vi "CLD3 FGV Timer Solution.vi"(8 "Fehler (Eingang)":T1, 10 "Zielzeit (s)":dbl, 11 "Timer-Modus":T2) -> (0 "Fehler (Ausgang)":T1, 2 "Zeit ist verstrichen":bool, 3 "Verstrichene Zeit (s,ms)":dbl format="%#.2f")   [LabVIEW 2009]
doc: "CLD-Übung 3\nDieses VI wird als FGV zum Messen von Zeit verwendet. \nHinweis zum Auslesen der Zeit während der Pause. Der Entwickler sollte die Funktion \"Zeit lesen\" nicht während der Pause aufrufen. Mit Hilfe einer Case-Struktur kann \"Status abfragen\" jedoch präventiv für diese Möglichkeit programmiert werden."
uses:
  CLD3 FGV Mode.ctl
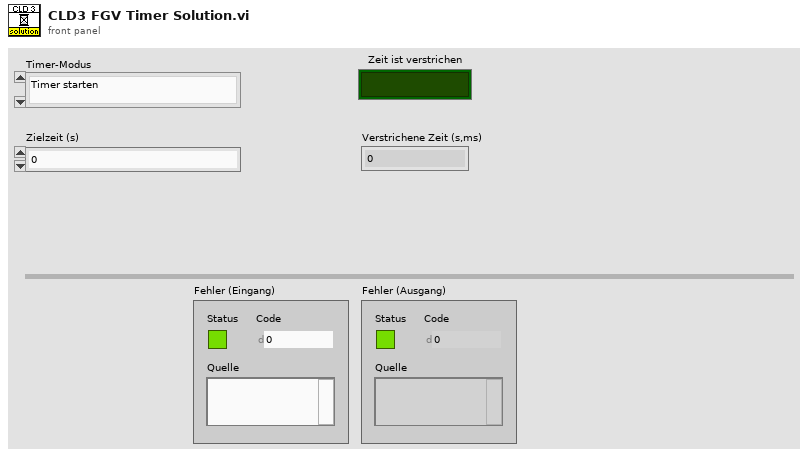
[diagram p1: front panel]
types:
  T1 = cluster{"Status":bool, "Code":i32, "Quelle":string}
  T2 = typedef "CLD3 FGV Mode.ctl" = enum16{"Timer starten", "Zeit lesen", "Anhalten", "Fortsetzen"}
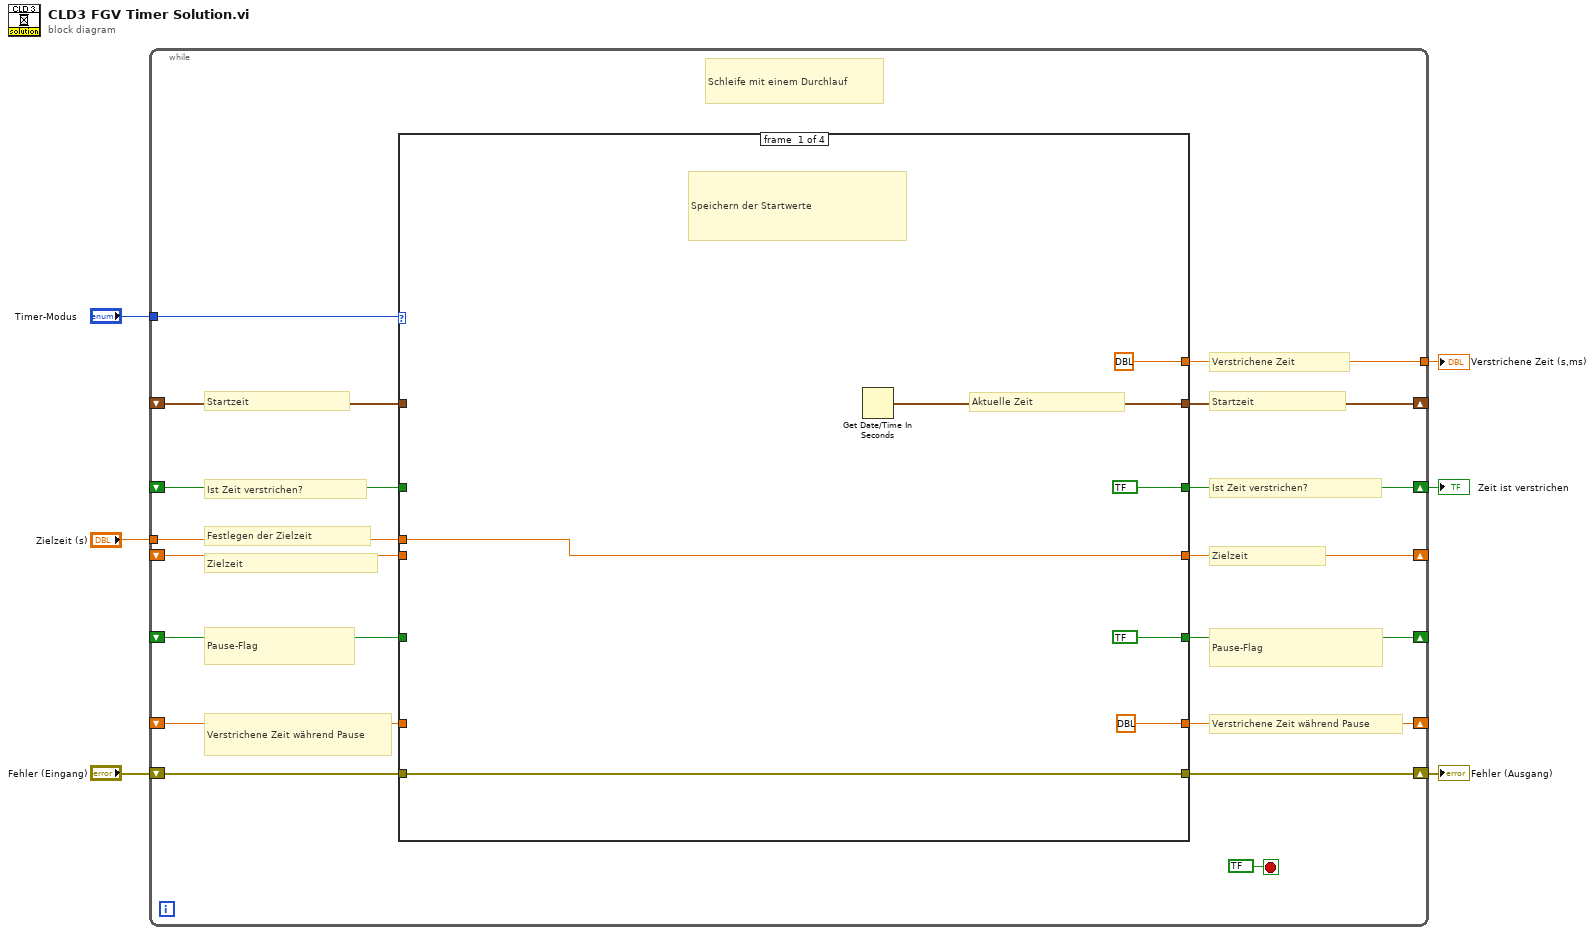
[diagram p0: block diagram]
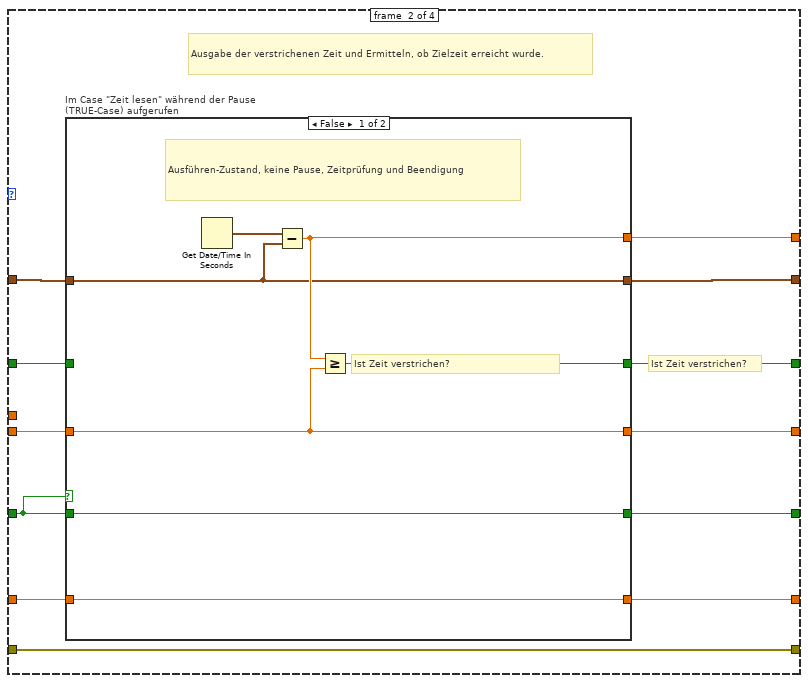
[diagram p2: hidden frame]
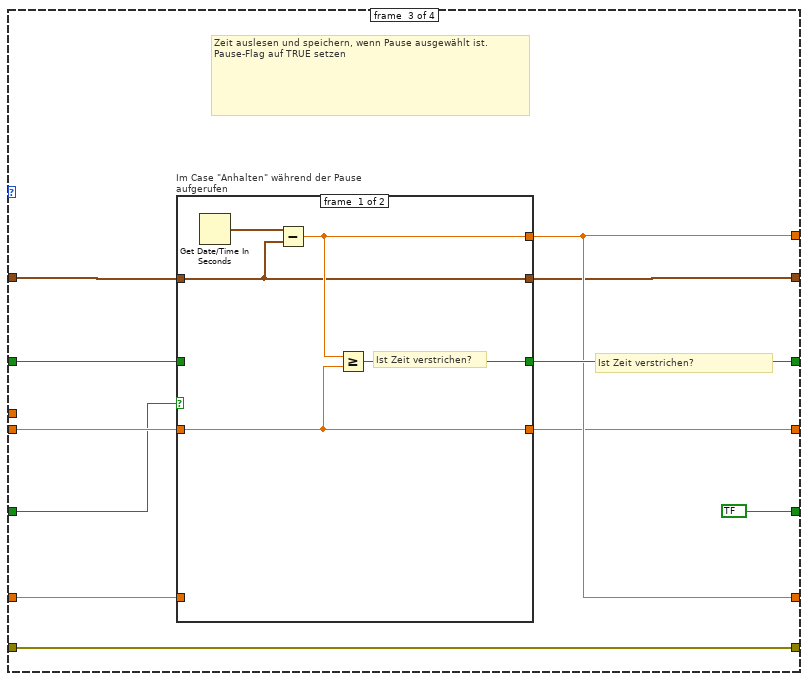
[diagram p4: hidden frame]
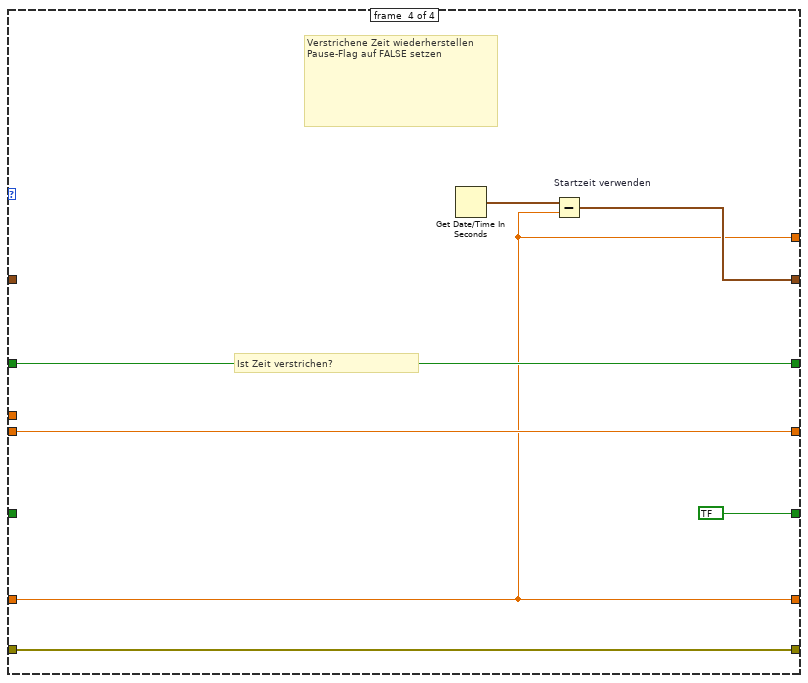
[diagram p6: hidden frame]
diagram:
  n1 = while {
    tunnel: "Timer-Modus" -> [w22]
    shift-right: [w20] -> _
    shift-left: _ -> [w19]
    tunnel: [w18] -> w1
    shift-right: [w17] -> w5
    shift-left: "Fehler (Eingang)" -> [w16]
    tunnel: "Zielzeit (s)" -> [w13]
    shift-right: [w14] -> _
    shift-left: _ -> [w15]
    shift-right: [w12] -> w2
    shift-left: _ -> [w11]
    shift-right: [w10] -> _
    shift-left: _ -> [w9]
    shift-right: [w8] -> _
    shift-left: _ -> [w7]
    stop <- bool ? ("Stopp") stop-if-true
    # "Startzeit"
    # "Startzeit"
    # "Verstrichene Zeit"
    # "Zielzeit"
    # "Zielzeit"
    # "Festlegen der Zielzeit"
    # "Ist Zeit verstrichen?"
    # "Ist Zeit verstrichen?"
    # "Pause-Flag"
    # "Pause-Flag"
    # "Verstrichene Zeit während Pause"
    # "Verstrichene Zeit während Pause"
    # "Schleife mit einem Durchlauf"
    n2 = case shown="\"Fortsetzen\"" w22 {
      tunnel: [w29 w33 w53 w74] -> w20
      tunnel: w19 -> [_ w40 w63 _]
      tunnel: [dbl ? ("Verstrichene Zeit") w36 w58 w73] -> w18
      tunnel: [w27 w39 w62 w79] -> w17
      tunnel: w16 -> [w27 w39 w62 w79]
      tunnel: w15 -> [_ w38 w61 w78]
      tunnel: [w26 w38 w54 w78] -> w14
      tunnel: w13 -> [w26 _ _ _]
      tunnel: [bool ? w37 w60 w76] -> w12
      tunnel: w11 -> [_ w30 w57 w76]
      tunnel: [bool ? w32 bool ? bool ?] -> w10
      tunnel: w9 -> [_ w31 w56 _]
      tunnel: [dbl ? w34 w58 w73] -> w8
      tunnel: w7 -> [_ w35 w55 w73]
      frame #0 {
        # "Aktuelle Zeit"
        # "Speichern der Startwerte"
        n3 = Get Date/Time In Seconds() -> (seconds since 1Jan1904=w29:timestamp)
      }
      frame #1 {
        # "Ist Zeit verstrichen?"
        # "Ausgabe der verstrichenen Zeit und Ermitteln, ob Zielzeit erreicht wurde."
        n4 = case "Im Case \"Zeit lesen\" während der Pause (TRUE-Case) aufgerufen" shown="False" w31 {
          tunnel: w40 -> [w44 w52]
          tunnel: w38 -> [w43 w51]
          tunnel: [w46 w49] -> w37
          tunnel: [w45 w48] -> w36
          tunnel: w35 -> [w41 w48]
          tunnel: [w41 w48] -> w34
          tunnel: [w44 w52] -> w33
          tunnel: [w43 w51] -> _
          tunnel: [w42 w50] -> w32
          tunnel: w31 -> [w42 w50]
          tunnel: w30 -> [_ w49]
          frame #0 {
            # "Ist Zeit verstrichen?"
            # "Ausführen-Zustand, keine Pause, Zeitprüfung und Beendigung"
            n5 = Get Date/Time In Seconds() -> (seconds since 1Jan1904=w47:timestamp)
            n6 = Subtract(x=w47, y=w44) -> (x-y=w45:dbl)
            n7 = Greater Or Equal?(x=w45, y=w43) -> (x >= y?=w46:bool)
          }
          frame #1 {
            # "Pause-Zustand, nur Ausgabe von Schieberegistern. \"Zeit lesen\" nicht während der Pause aufrufen."
          }
        }
      }
      frame #2 {
        # "Ist Zeit verstrichen?"
        # "Zeit auslesen und speichern, wenn Pause ausgewählt ist.\nPause-Flag auf TRUE setzen"
        n8 = case "Im Case \"Anhalten\" während der Pause aufgerufen" shown="True" w56 {
          tunnel: w63 -> [w64 w69]
          tunnel: w61 -> [w65 w70]
          tunnel: [w67 w72] -> w60
          tunnel: [w66 w71] -> w58
          tunnel: w57 -> [_ w72]
          tunnel: w55 -> [_ w71]
          tunnel: [w65 w70] -> w54
          tunnel: [w64 w69] -> w53
          frame #0 {
            # "Ist Zeit verstrichen?"
            n9 = Get Date/Time In Seconds() -> (seconds since 1Jan1904=w68:timestamp)
            n10 = Subtract(x=w68, y=w64) -> (x-y=w66:dbl)
            n11 = Greater Or Equal?(x=w66, y=w65) -> (x >= y?=w67:bool)
          }
          frame #1 {
            # "Pause wurde während der Pause aufgerufen.\n\nNur Schieberegister auslesen und Werte weitergeben."
          }
        }
      }
      frame #3 {
        # "Ist Zeit verstrichen?"
        # "Verstrichene Zeit wiederherstellen\nPause-Flag auf FALSE setzen"
        n12 = Get Date/Time In Seconds() -> (seconds since 1Jan1904=w75:timestamp)
        n13 = Subtract "Startzeit verwenden"(x=w75, y=w73) -> (x-y=w74:timestamp)
      }
    }
  }
  "Fehler (Ausgang)" <- w5
  "Zeit ist verstrichen" <- w2
  "Verstrichene Zeit (s,ms)" <- w1
